vi "Log Message to the Caller.vi"(6 "String (\"\" = no message to send)":string, 8 "error in (no error)":errorcluster, 11 "CO2 Actor in":refnum<class "CO2 Actor.lvclass">) -> (0 "error out":errorcluster, 3 "CO2 Actor out":refnum<class "CO2 Actor.lvclass">)   [LabVIEW 2015, in "cRIO-Carbondioxide.lvlib" / "CO2-Actor.lvlib" / "CO2 Actor.lvclass"]
uses:
  CO2 Actor.lvclass
  CO2 Actor.lvclass/CO2 Actor.ctl
  <vilib>/ActorFramework/Message Enqueuer/Message Priority.ctl
  cRIO-CO2 Messages/Log Message Msg/Log Message Msg.lvclass/Log Message Msg.ctl
  <vilib>/ActorFramework/Message Enqueuer/Message Enqueuer.lvclass/Message Enqueuer.ctl
  <vilib>/ActorFramework/Message Enqueuer/Enqueue.vi
  <vilib>/ActorFramework/Message Priority Queue/Priority Enqueue.vi
  cRIO-CO2 Messages/Log Message Msg/Log Message Msg.lvclass
  <vilib>/ActorFramework/Message Enqueuer/Message Enqueuer.lvclass
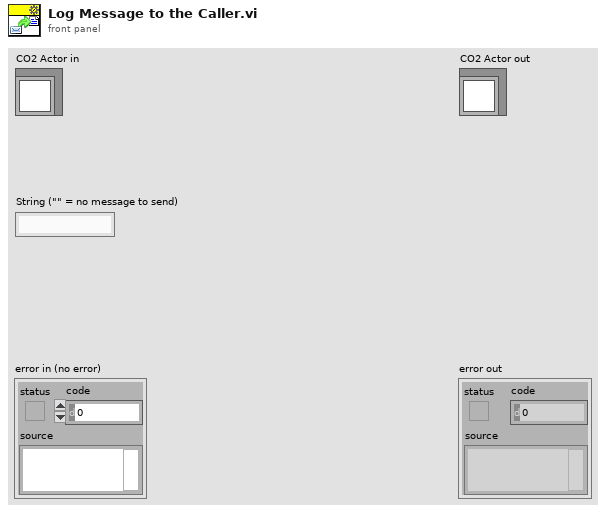
[diagram p1: front panel]
types:
  T1 = typedef "Actor Framework.lvlib/Message Enqueuer.lvclass/Message Priority.ctl" = enum16{"Low", "Normal", "High"}
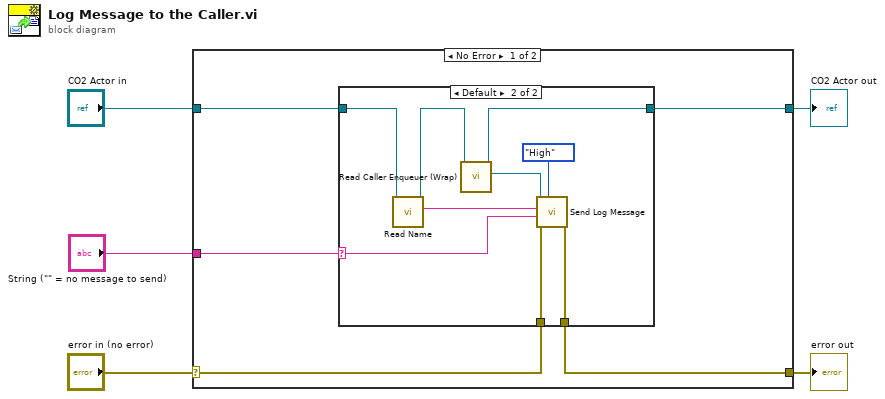
[diagram p0: block diagram]
diagram:
  n1 = case shown="No Error" "error in (no error)" {
    selector: "error in (no error)" -> [w10 w23]
    tunnel: [w9 w23] -> w4
    tunnel: [w6 w22] -> w2
    tunnel: "CO2 Actor in" -> [w7 w22]
    tunnel: "String (\"\" = no message to send)" -> [w8 _]
    frame No Error {
      n2 = case shown="Default" w8 {
        selector: w8 -> [_ w17]
        tunnel: w10 -> [w11 w19]
        tunnel: [w11 w18] -> w9
        tunnel: w7 -> [w12 w16]
        tunnel: [w12 w14] -> w6
        frame "" {
        }
        frame Default {
          n3 = call "Read Name.vi"("CO2 Actor in"=w16) -> ("Name"=w21:string, "CO2 Actor out"=w15:refnum<class "CO2 Actor.lvclass">)  [unwired: 9 in]
          n4 = call "Read Caller Enqueuer (Wrap).vi"("CO2 Actor in"=w15) -> ("Actor Framework:Message Enqueuer"=w20:refnum<class "Message Enqueuer.lvclass">, "CO2 Actor out"=w14:refnum<class "CO2 Actor.lvclass">)  [unwired: 9 in]
          n5 = call "Send Log Message.vi"("Message Priority (Normal)"=Message_Priority."High", "error in (no error)"=w19, "String"=w17, "Source Name"=w21, "Message Enqueuer"=w20) -> ("error out"=w18:errorcluster)  [unwired: 5 in, 1 out]
        }
      }
    }
    frame Error {
    }
  }
  "error out" <- w4
  "CO2 Actor out" <- w2
